vi "Main.vi"() -> ()   [LabVIEW 2012]
uses:
  HeaterConfigurationGlobalAction.ctl
  MFCConfigurationGlobalAction.ctl
  LogActionQueueElement.ctl
  LogAction.ctl
  HardwareActionQueueElement.ctl
  HardwareAction.ctl
  HeaterActionQueueElement.ctl
  HeaterAction.ctl
  MFCActionQueueElement.ctl
  MFCAction.ctl
  <vilib>/Utility/error.llb/DialogType.ctl
  UIActionQueueElement.ctl
  UIAction.ctl
  libs/LV-Utilities/LV-Utilities.lvlib
panel:
  in  "LOGS":bool
  in  "LIVE":bool
  in  "SYSTEM":bool
  in  "DONE":bool
  in  "Tab Control":enum32{"System", "Live", "Logs"}(tab)
  out "MFC Serial Number":string="Serial Number"
  in  "SELECT CONFIG":bool
  out "Setup File":path
  in  "CONFIGURE MFC":bool
  in  "CONFIGURE HEATER":bool
  out "Chamber Name":string="Chamber Name"
  out "Heater Actual Slide":dbl(slide) scale=0.0..200.0 scale format="%#.1f"
  out "Heater Actual (C)":dbl=nan format="%.1f"
  out "Heater Setpoint Slide":dbl(slide) scale=0.0..200.0 scale format="%#.1f"
  out "Heater Setpoint (C)":dbl=nan format="%.1f"
  out "Heater State":enum16{"Not Connected", "Run", "Standby"}(ring)
  out "MFC Actual Slide":dbl(slide) scale=0.0..1000.0 scale format="%#.1f"
  out "MFC Actual (mL/min)":dbl=nan format="%.1f"
  out "MFC Setpoint Slide":dbl(slide) scale=0.0..1000.0 scale format="%#.1f"
  out "MFC Setpoint (mL/min)":dbl=nan format="%.1f"
  out "MFC Valve State":T1(ring)
  out "Live Heater Chart":cluster{"Setpoint (C)":dbl, "Actual (C)":dbl}(graph)
  out "Live MFC Chart":T2(graph)
  in  "CLEAR CHARTS":bool
  out "Heater Setpoint Chart (C)":dbl=nan format="%.1f"
  out "Heater Actual Chart (C)":dbl=nan format="%.1f"
  out "MFC Setpoint Chart (mL/min)":dbl=nan format="%.1f"
  out "MFC Actual Chart (mL/min)":dbl=nan format="%.1f"
  out "MFC Graph":cluster{timestamp[], "Y Data":dbl[]}[](graph)
  out "Heater Graph":cluster{timestamp[], "Y Data":dbl[]}[](graph)
  in  "OPEN LOG":bool
  in  "CLOSE LOG":bool
  out "Opened Log File Path":path
  # "Vacuum Pump"
  # "Config File:"
  # "Actual"
  # "Setpoint"
  # "Actual"
  # "Setpoint"
  # "Heater:"
  # "MFC:"
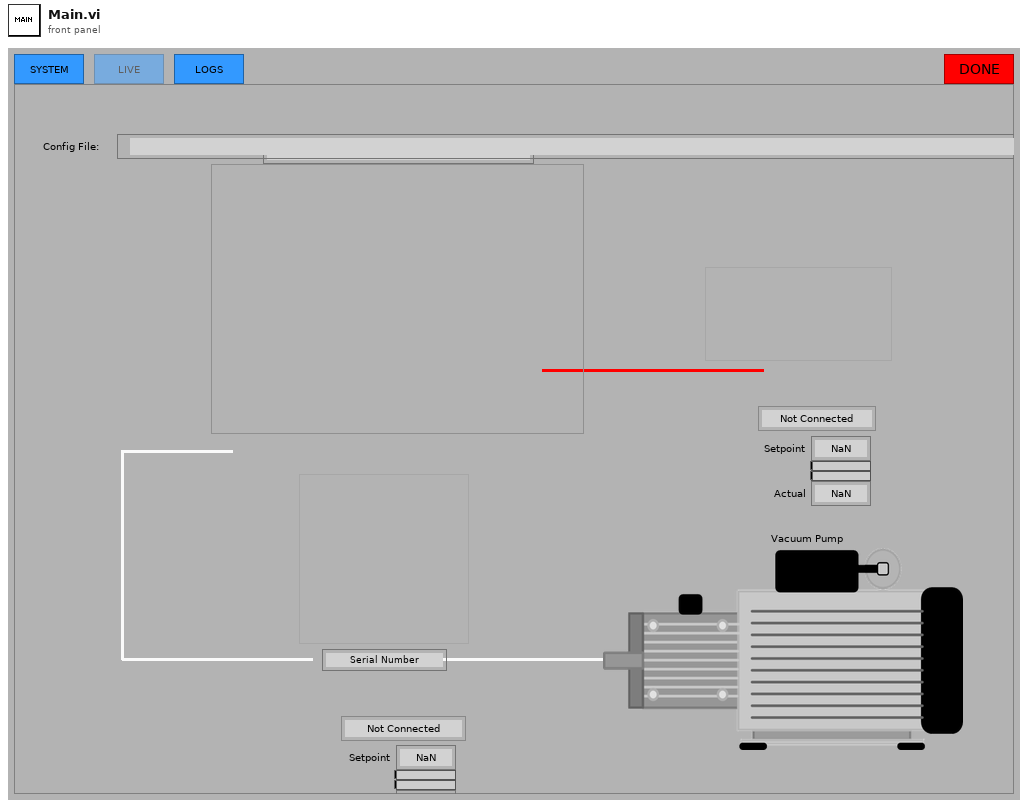
[diagram p1: front panel]
types:
  T1 = enum16{"Not Connected", "Automatic", "Closed", "Purge"}
  T2 = cluster{"Setpoint (mL/min)":dbl, "Actual (mL/min)":dbl}
  T3 = typedef "DataStructures.ctl" = cluster{"Display":refnum<notifier>, "Log":refnum<queue>}
  T4 = typedef "ActionQueues.ctl" = cluster{"UI Action":refnum<queue>, "Hardware Action":refnum<queue>, "Heater Action":refnum<queue>, "MFC Action":refnum<queue>, "Log Action":refnum<queue>}
  T5 = typedef "ExecutableConfiguration.ctl" = cluster{"Default Chamber Folder Path":path, "Default Log Folder Path":path, "Default Monitor":i32, "Center on Monitor?":bool}
  T6 = typedef "MFCActionQueueElement.ctl" = cluster{"Action":T7, "Data":variant}
  T7 = typedef "MFCAction.ctl" = enum16{"Initialize", "Start", "Read", "Write", "Stop", "Error", "Shutdown"}
  T8 = typedef "HeaterActionQueueElement.ctl" = cluster{"Action":T9, "Data":variant}
  T9 = typedef "HeaterAction.ctl" = enum16{"Initialize", "Start", "Read", "Write", "Stop", "Error", "Shutdown"}
  T10 = typedef "HardwareActionQueueElement.ctl" = cluster{"Action":T11, "Data":variant}
  T11 = typedef "HardwareAction.ctl" = enum16{"Initialize", "Collect", "Shutdown"}
  T12 = enum8{"Enabled", "Disabled", "Disabled and Grayed Out"}
  T13 = typedef "LogActionQueueElement.ctl" = cluster{"Action":T14, "Data":variant}
  T14 = typedef "LogAction.ctl" = enum16{"Initialize", "Start", "Log", "Stop", "Error", "Shutdown"}
  T15 = typedef "MFCConfigurationGlobalAction.ctl" = enum16{"Get", "Set", "Reset"}
  T16 = typedef "HeaterConfigurationGlobalAction.ctl" = enum16{"Get", "Set", "Reset"}
  T17 = cluster{"Setpoint (mL/min)":dbl, "Actual (mL/min)":dbl}[]
  T18 = typedef "UIActionQueueElement.ctl" = cluster{"Action":T19, "Data":variant}
  T19 = typedef "UIAction.ctl" = enum16{"Initialize", "Connect", "MFC Connected", "Heater Connected", "Disconnect", "MFC Disconnected", "Heater Disconnected", "Configure MFC", "Configure Heater", "Open Log", "Close Log", "Shutdown"}
  T20 = typedef "Setup.ctl" = cluster{"Chamber Name":string, "Log Folder Path":path, "Heater":T21, "MFC":T22}
  T21 = typedef "HeaterConfiguration.ctl" = cluster{"COM Port":u8, "Setpoint":dbl, "Standby?":bool}
  T22 = typedef "MFCConfiguration.ctl" = cluster{"COM Port":u32, "Timeout (msec)":u32, "Setpoint":dbl, "Valve State":T23, "Gas":T24, "Units":T25, "Serial Number":string, "Firmware Version":string}
  T23 = typedef "Sierra-M100.lvlib/ValveState.ctl" = enum16{"Automatic", "Closed", "Purge"}
  T24 = typedef "Sierra-M100.lvlib/Gas.ctl" = enum16{"Air", "Argon", "CO2", "CO", "Helium", "Hydrogen", "Methane", "Nitrogen", "Nitrous Oxide", "Oxygen"}
  T25 = typedef "Sierra-M100.lvlib/Units.ctl" = enum16{"scc/s", "scc/m", "scc/H", "Ncc/s", "Ncc/m", "Ncc/H", "SCF/s", "SCF/m", "SCF/H", "NM3/s", "NM3/m", "NM3/H", "SM3/s", "SM3/m", "SM3/H", "sl/s", "sl/m", "sl/H", "NL/s", "NL/m", "Nl/H", "g/s", "g/m", "g/H", "kg/s", "kg/m", "kg/H", "lb/s", "lb/m", "lb/H"}
  T26 = typedef "DialogType.ctl" = u16
  T27 = typedef "HardwareDisplayData.ctl" = cluster{"Heater":dbl, "MFC":dbl}
  T28 = typedef "MFCDisplayValveState.ctl" = enum16{"Not Connected", "Automatic", "Closed", "Purge"}
  T29 = typedef "HeaterDisplayState.ctl" = enum16{"Not Connected", "Run", "Standby"}
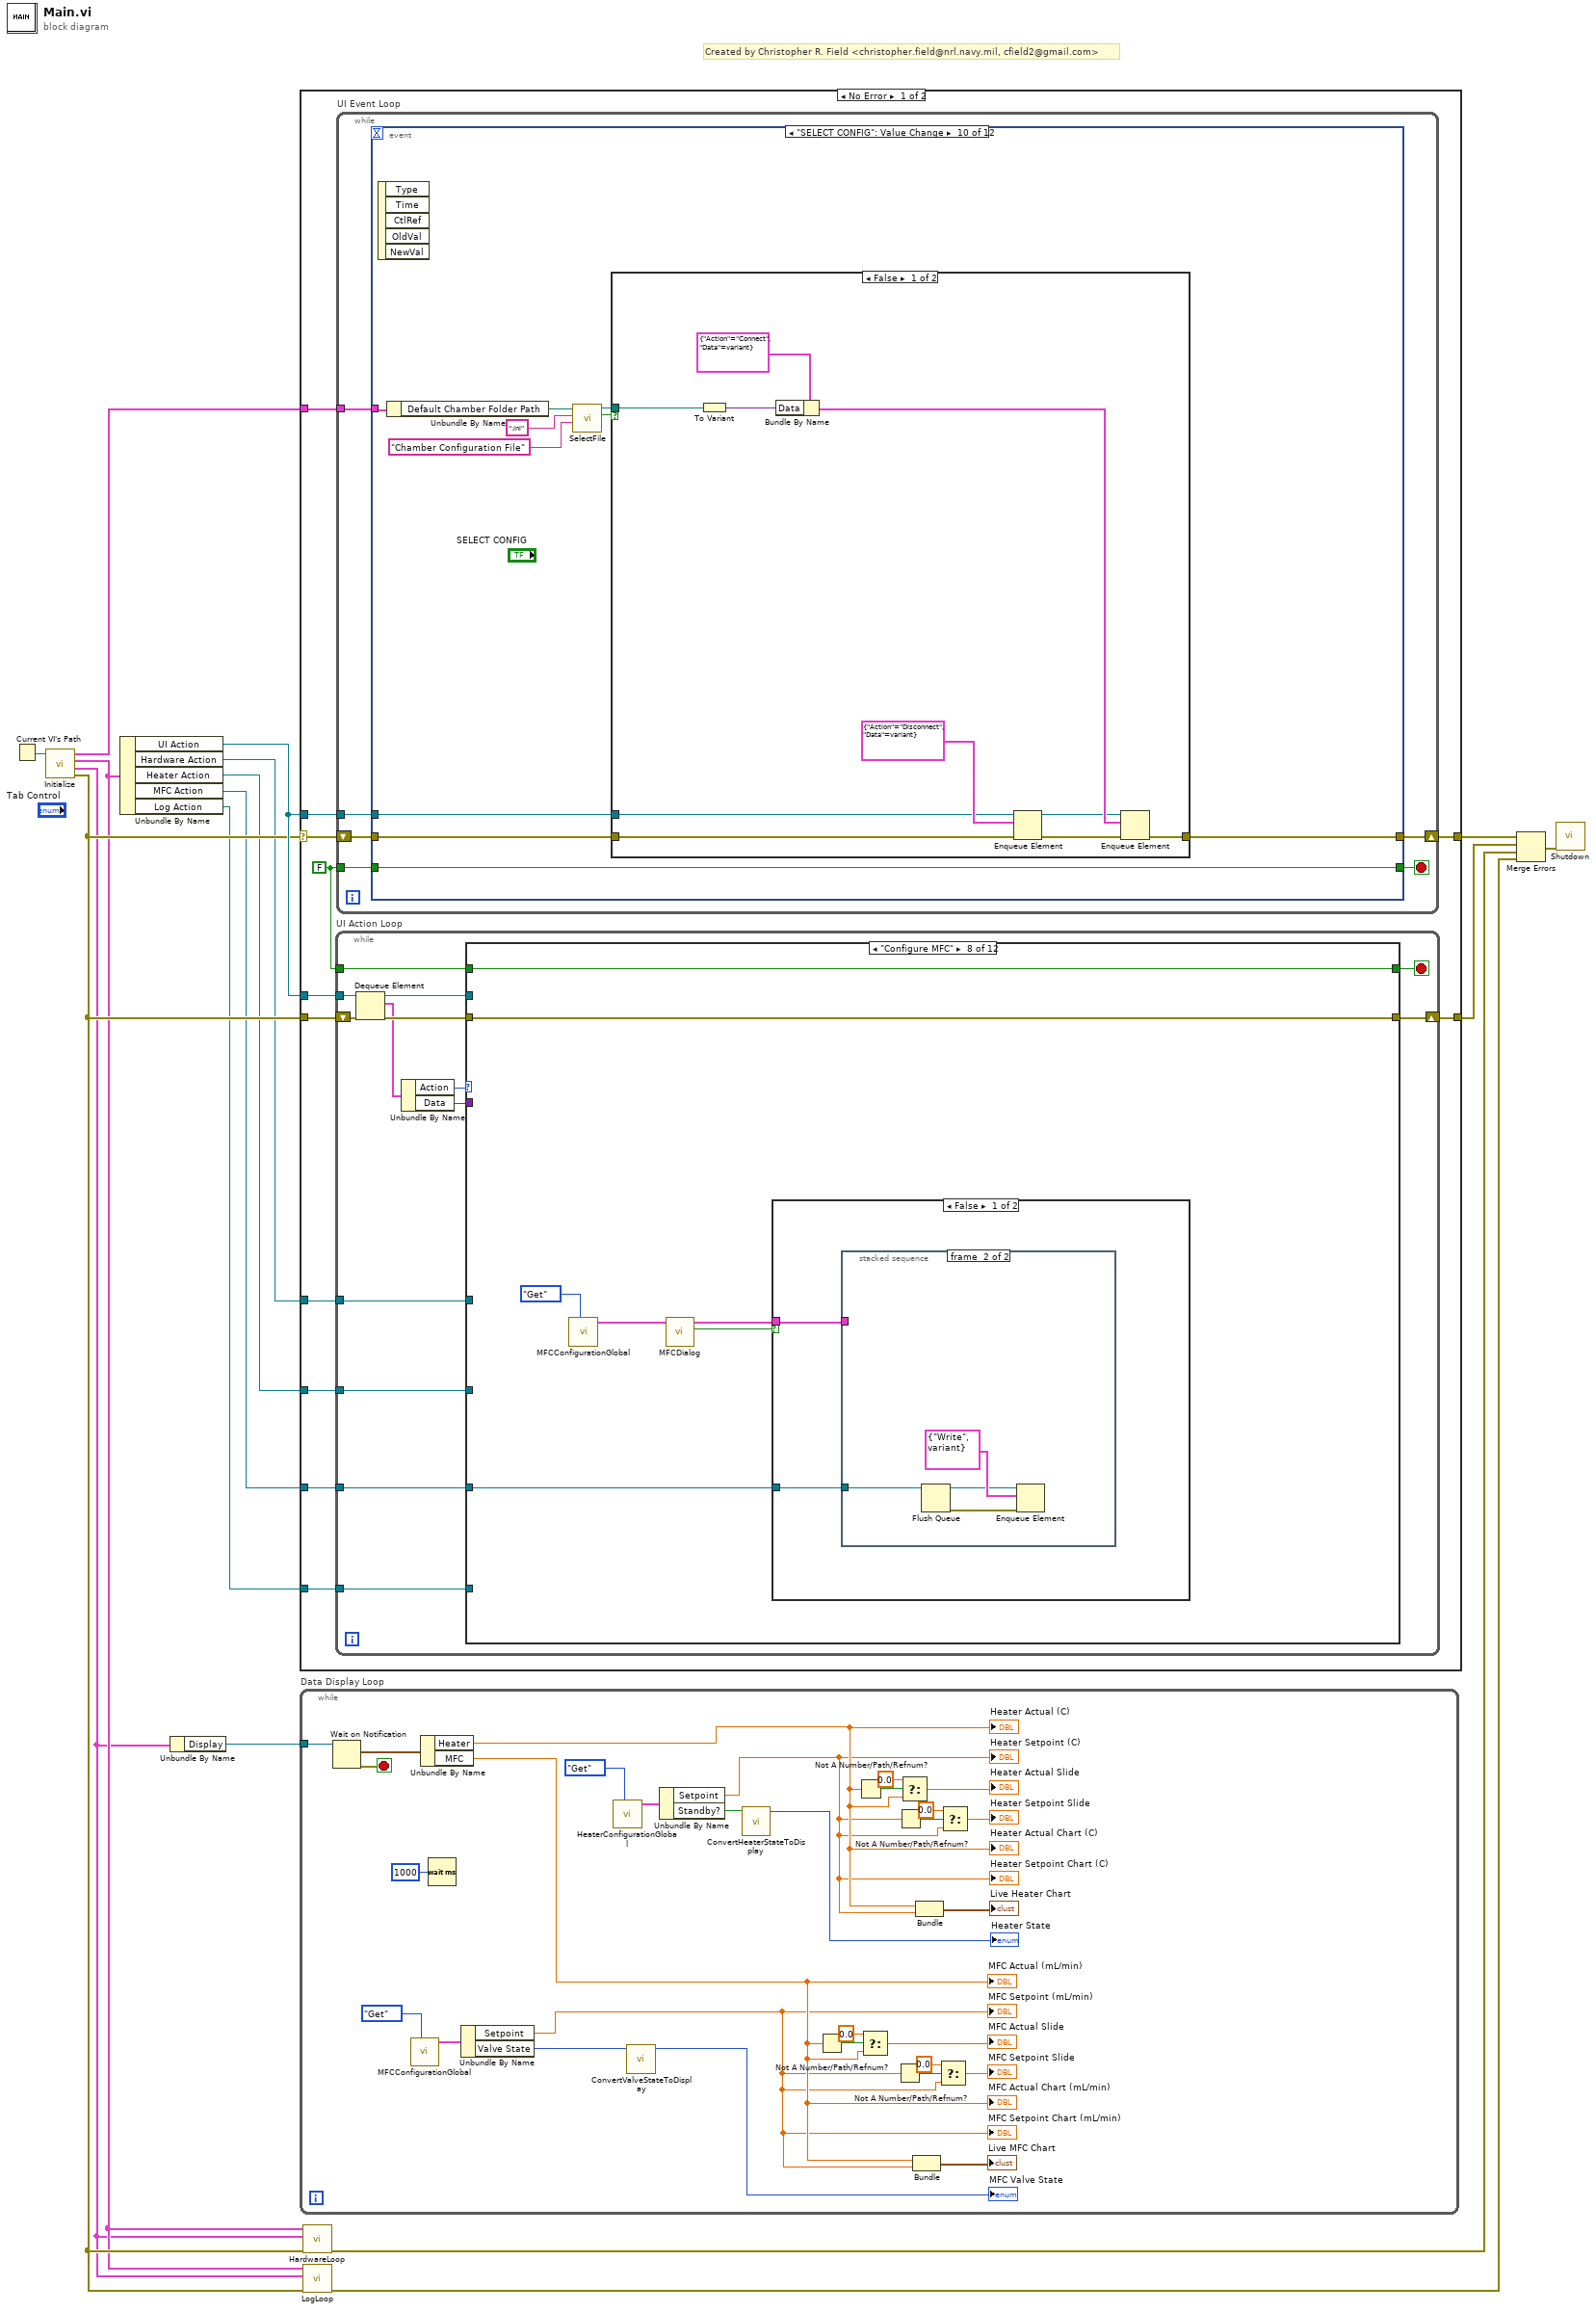
[diagram p0: block diagram]
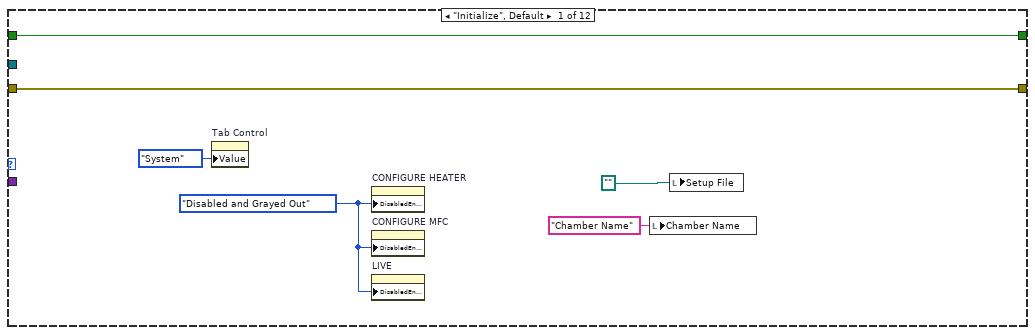
[diagram p2: hidden frame]
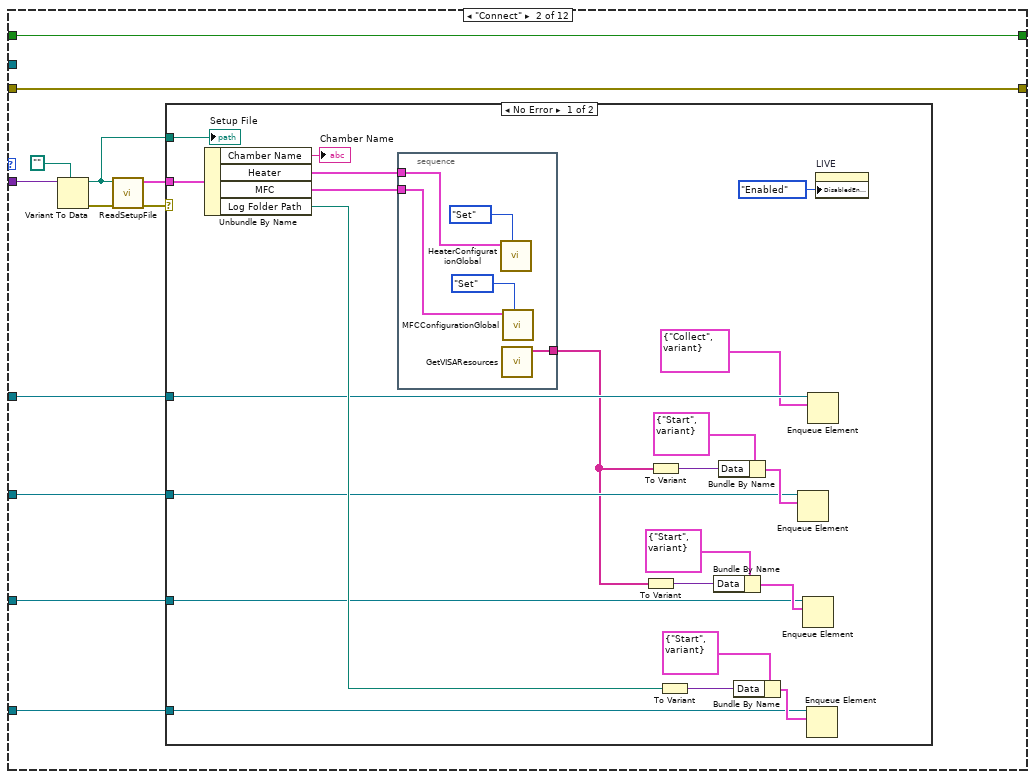
[diagram p3: hidden frame]
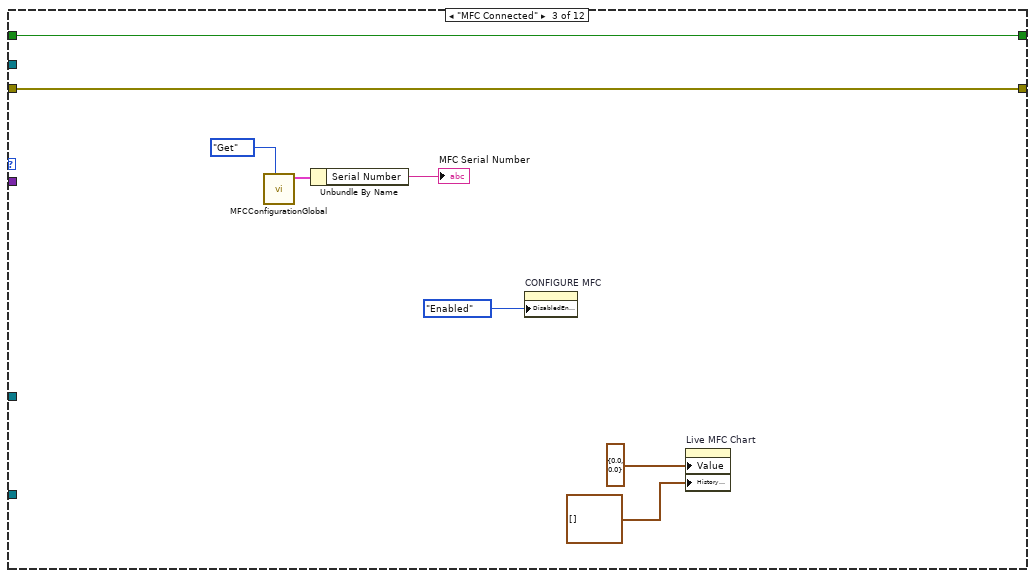
[diagram p5: hidden frame]
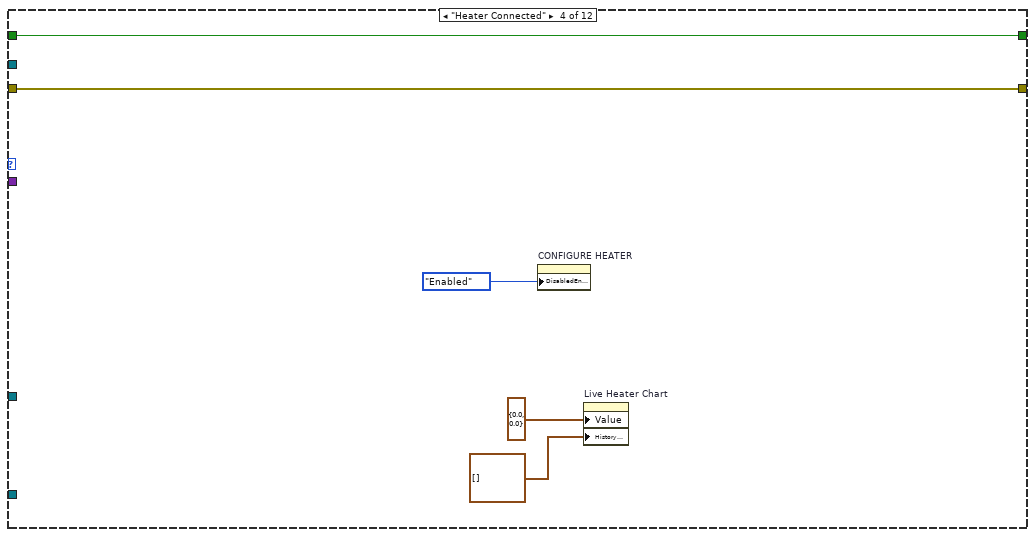
[diagram p6: hidden frame]
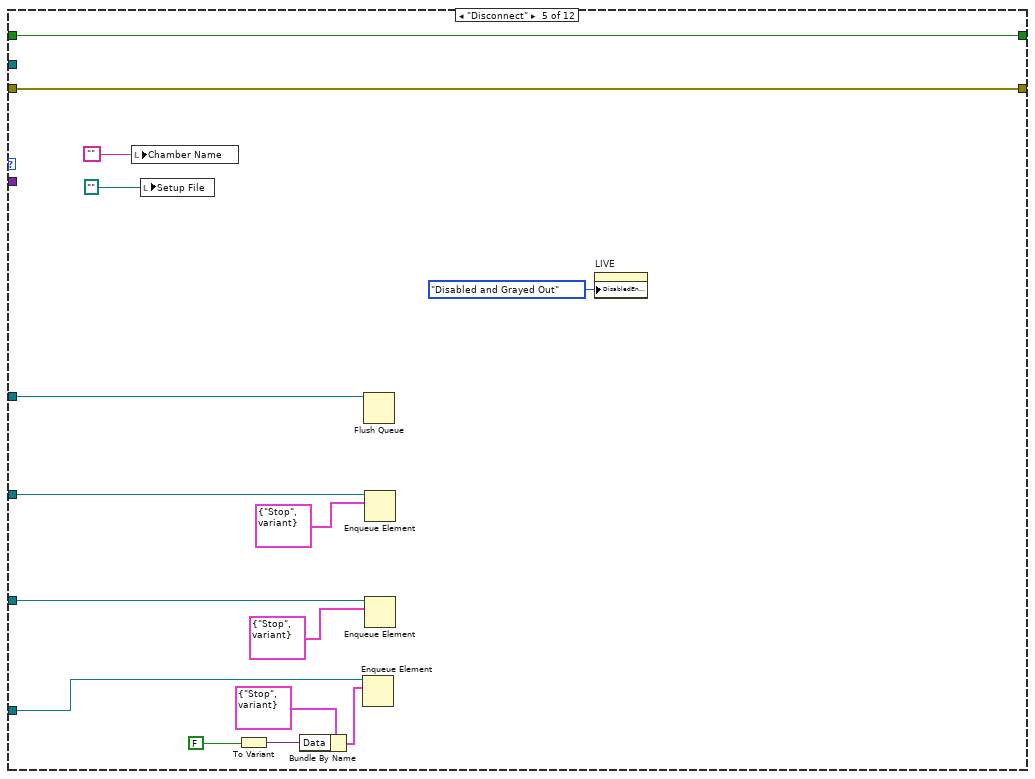
[diagram p7: hidden frame]
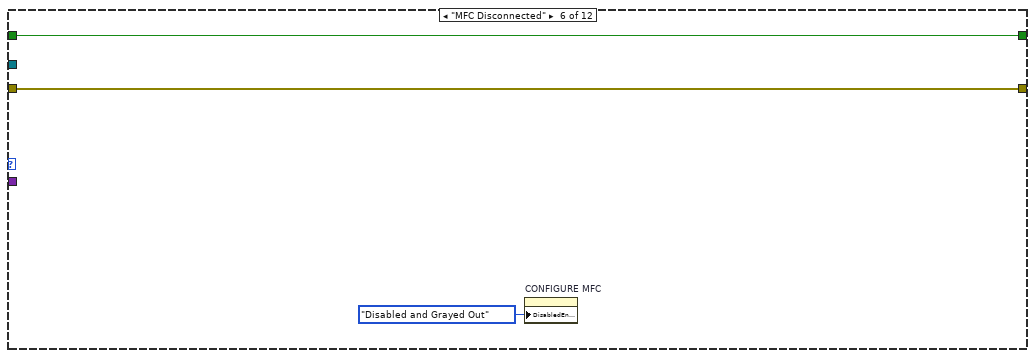
[diagram p8: hidden frame]
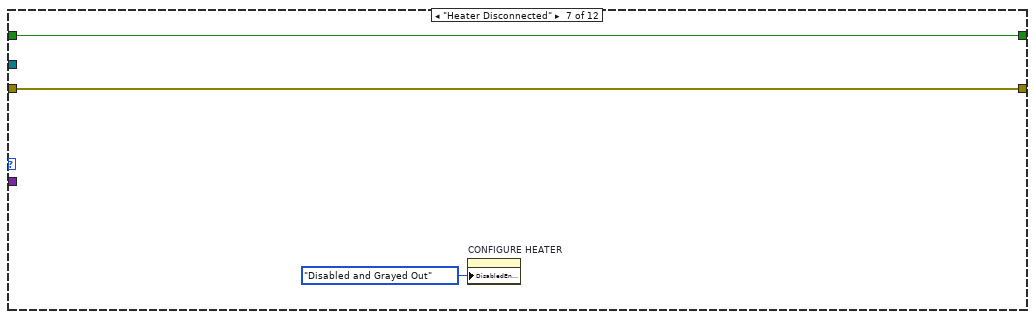
[diagram p9: hidden frame]
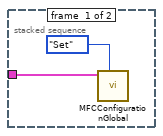
[diagram p10: hidden frame]
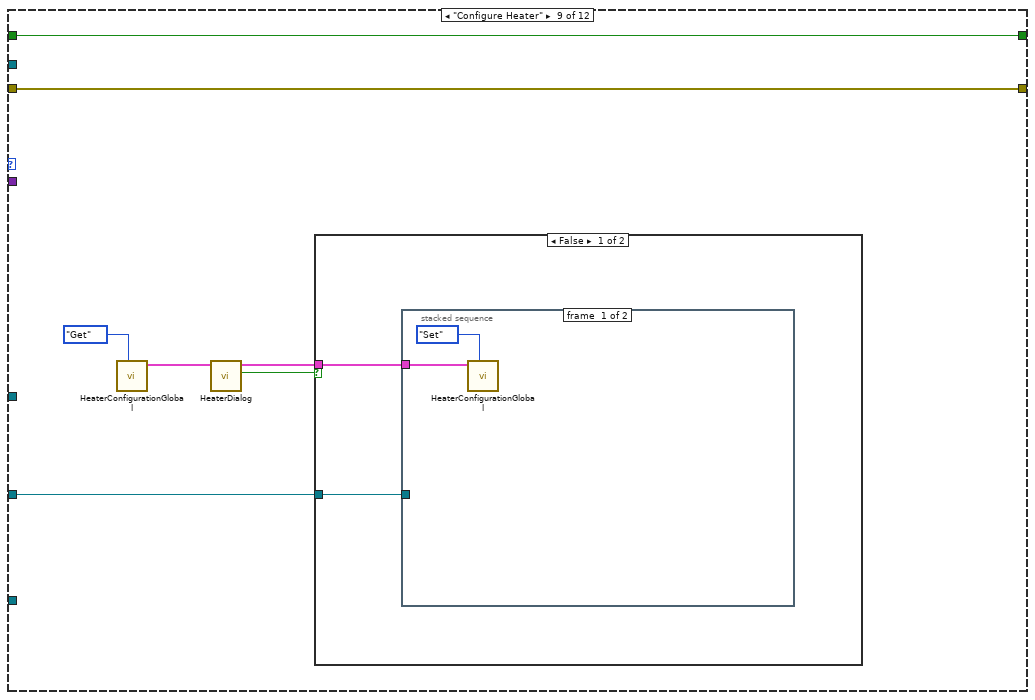
[diagram p12: hidden frame]
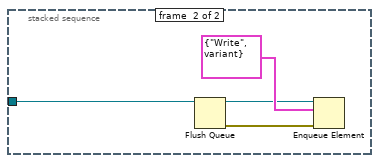
[diagram p13: hidden frame]
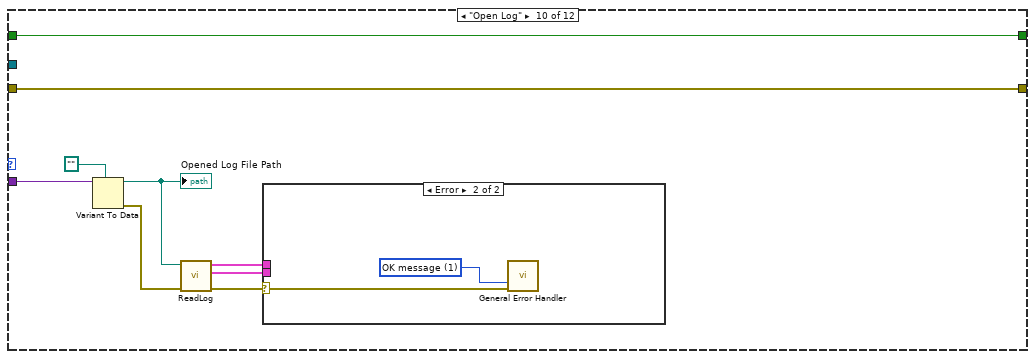
[diagram p15: hidden frame]
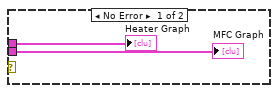
[diagram p16: hidden frame]
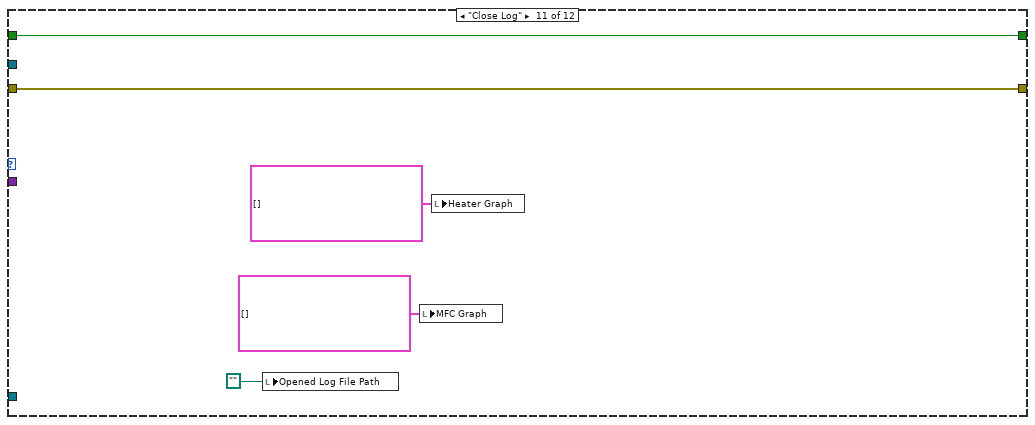
[diagram p17: hidden frame]
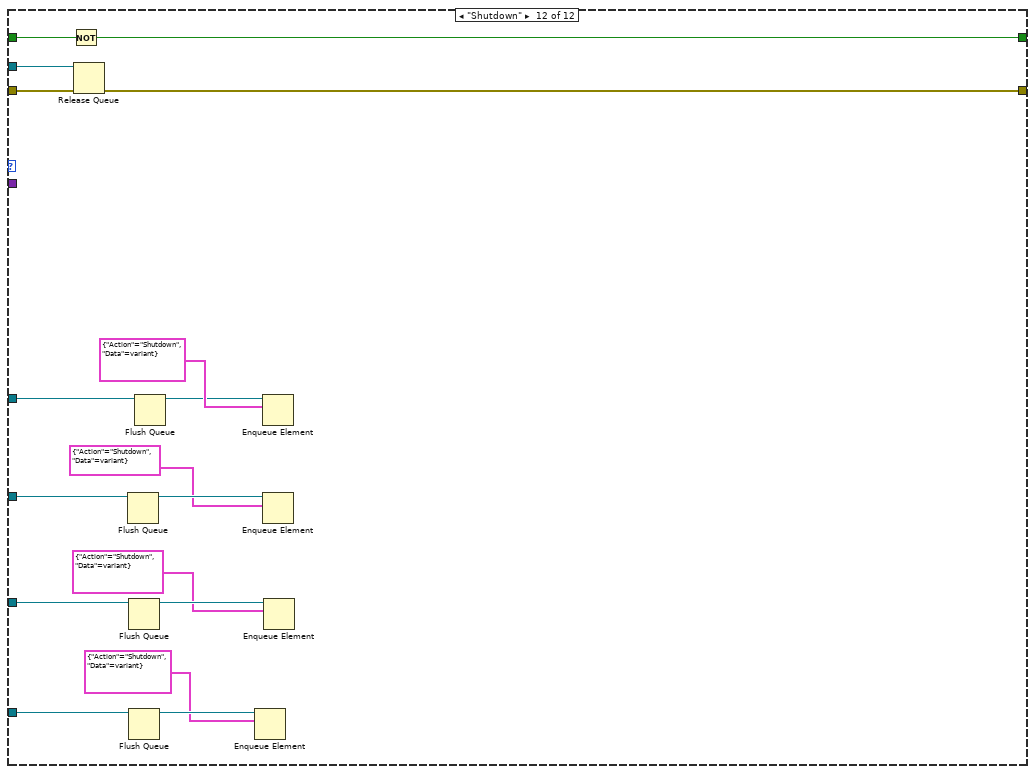
[diagram p18: hidden frame]
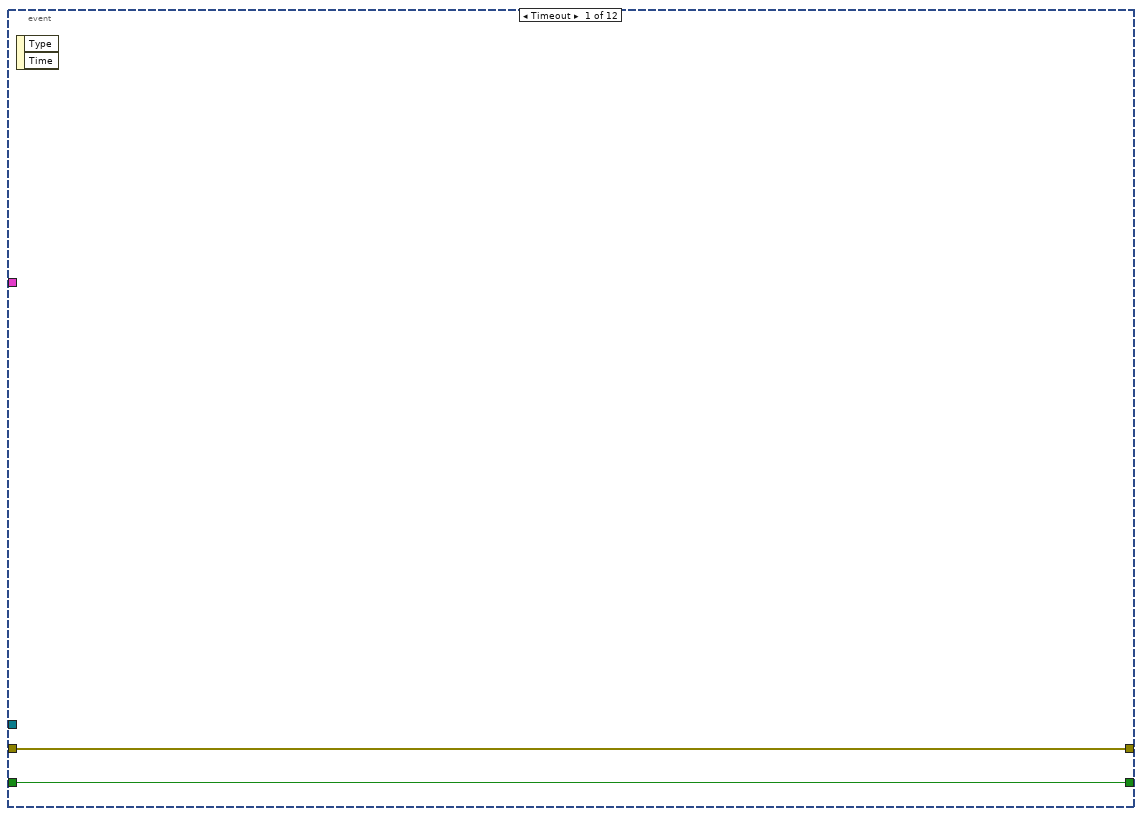
[diagram p19: hidden frame]
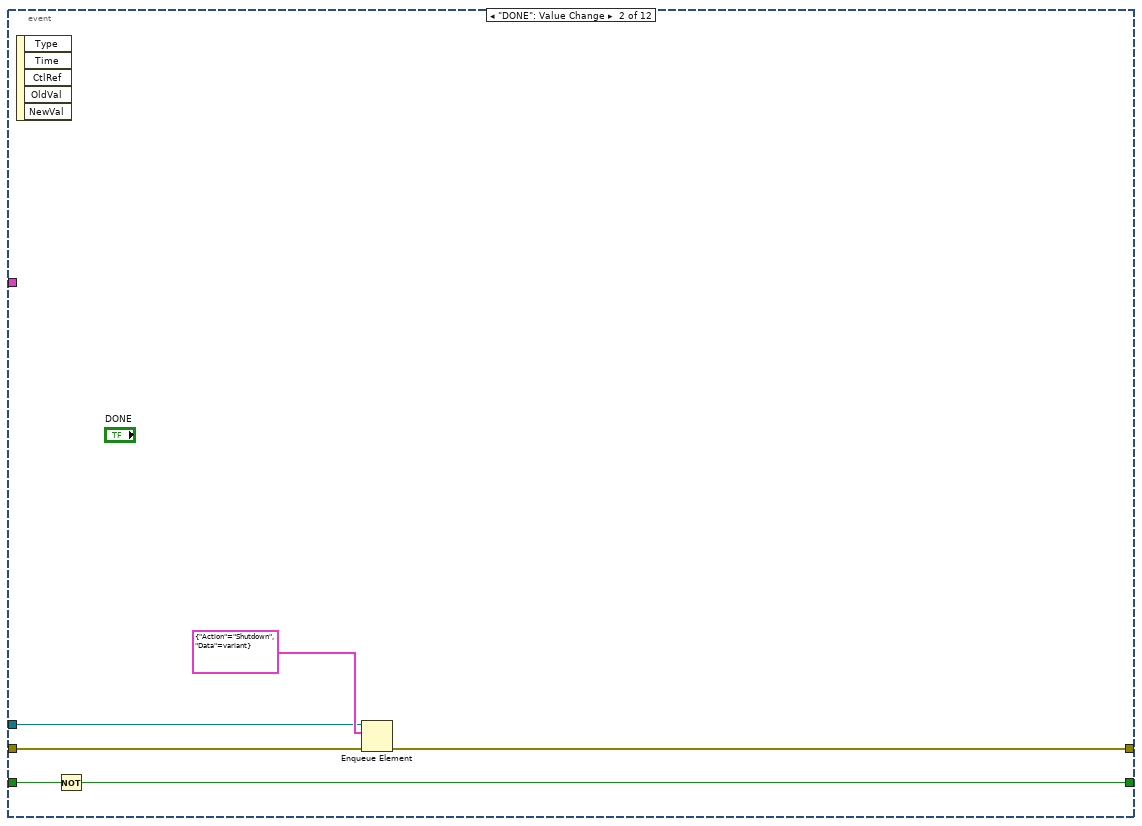
[diagram p20: hidden frame]
diagram:
  # "Created by Christopher R. Field <christopher.field@nrl.navy.mil, cfield2@gmail.com>"
  n1 = Current VI's Path() -> (path=w16:path)
  n2 = call "Initialize.vi"("VI Path"=w16) -> ("Error Out"=w11:errorcluster, "Data Structures"=w6:T3, "Action Queues"=w7:T4, "Executable Configuration"=w4:T5)  [unwired: 7 in]
  n3 = Unbundle By Name(w7) -> ("UI Action"=w15:refnum<queue>, "Hardware Action"=w8:refnum<queue>, "Heater Action"=w3:refnum<queue>, "MFC Action"=w2:refnum<queue>, "Log Action"=w1:refnum<queue>)
  n4 = Unbundle By Name(w6) -> ("Display"=w5:refnum<notifier>)
  n5 = case shown="No Error" w11 {
    selector: w11 -> [w27 w277]
    tunnel: [w28 w277] -> w14
    tunnel: w15 -> [w25 _]
    tunnel: w11 -> [w24 w276]
    tunnel: w15 -> [w23 _]
    tunnel: [w22 w276] -> w13
    tunnel: w8 -> [w21 _]
    tunnel: w4 -> [w20 _]
    tunnel: w3 -> [w19 _]
    tunnel: w2 -> [w18 _]
    tunnel: w1 -> [w17 _]
    frame No Error {
      w26 = FALSE
      n6 = while "UI Action Loop" {
        tunnel: w26 -> [w42]
        tunnel: w25 -> [w32]
        shift-right: [w35] -> w22
        shift-left: w24 -> [w41]
        tunnel: w21 -> [w33]
        tunnel: w19 -> [w31]
        tunnel: w18 -> [w30]
        tunnel: w17 -> [w29]
        stop <- w34 stop-if-true
        n7 = Dequeue Element(queue=w32, error in (no error)=w41) -> (queue out=w40:refnum<queue>, element=w38:T18, error out=w39:errorcluster)  [unwired: 1 in, 1 out]
        n8 = Unbundle By Name(w38) -> ("Action"=w37:T19, "Data"=w36:variant)
        n9 = case shown="\"Configure MFC\"" w37 {
          tunnel: w42 -> [w48 w60 w95 w99 w115 w118 w121 w128 w143 w160 w169 w186]
          tunnel: w40 -> [_ _ _ _ _ _ _ _ _ _ _ w184]
          tunnel: w39 -> [w47 w59 w94 w100 w114 w117 w120 w127 w142 w159 w168 w183]
          tunnel: w36 -> [_ w58 _ _ _ _ _ _ _ w158 _ _]
          tunnel: [w47 w59 w94 w100 w114 w117 w120 w127 w142 w159 w168 w182] -> w35
          tunnel: [w48 w60 w95 w99 w115 w118 w121 w128 w143 w160 w169 w185] -> w34
          tunnel: w33 -> [_ w52 _ _ w101 _ _ _ _ _ _ w171]
          tunnel: w31 -> [_ w51 _ _ w104 _ _ _ w141 _ _ w175]
          tunnel: w30 -> [_ w50 _ _ w103 _ _ w126 _ _ _ w174]
          tunnel: w29 -> [_ w49 _ _ w102 _ _ _ _ _ _ w173]
          frame "Initialize", Default {
            w45 = T12."Disabled and Grayed Out" ("Disabled")
            n10 = property on="Tab Control" class="TabCtl (strict)"("Value"=enum32{"System", "Live", "Logs"}."System" ("Tab Control")) -> ()  [unwired: 2 in, 2 out]
            n11 = property on="CONFIGURE HEATER" class="Bool"("DisabledEnum"=w45) -> ()  [unwired: 2 in, 2 out]
            n12 = property on="CONFIGURE MFC" class="Bool"("DisabledEnum"=w45) -> ()  [unwired: 2 in, 2 out]
            n13 = property on="LIVE" class="Bool"("DisabledEnum"=w45) -> ()  [unwired: 2 in, 2 out]
            n14 = local write "Chamber Name"("Chamber Name" ("Chamber Name")) -> ()
            n15 = local write "Setup File"(path "") -> ()
          }
          frame "Connect" {
            n16 = Variant To Data(type=path "", Variant=w58) -> (data=w53:path, error out=w56:errorcluster)  [unwired: 1 in]
            n17 = call "ReadSetupFile.vi"("Error In"=w56, "Setup File"=w53) -> ("Error Out"=w55:errorcluster, "Setup"=w54:T20)  [unwired: 8 in]
            n18 = case shown="No Error" w55 {
              tunnel: w54 -> [w82 _]
              tunnel: w53 -> [w80 _]
              tunnel: w52 -> [w74 _]
              tunnel: w51 -> [w67 _]
              tunnel: w50 -> [w66 _]
              tunnel: w49 -> [w64 _]
              frame No Error {
                n19 = Unbundle By Name(w82) -> ("Chamber Name"=→"Chamber Name":string, "Heater"=w63:T21, "MFC"=w62:T22, "Log Folder Path"=w77:path)
                n20 = stacked-sequence {
                  tunnel: w63 -> [w86]
                  tunnel: w62 -> [w85]
                  tunnel: [w83] -> w61
                  frame #0 {
                    n21 = call "HeaterConfigurationGlobal.vi"("Action"=HeaterConfigurationGlobalAction."Set", "Set Value"=w86) -> ()  [unwired: 9 in, 1 out]
                    n22 = call "GetVISAResources.vi"() -> ("VISA Resources"=w83:string[])  [unwired: 10 in, 1 out]
                    n23 = call "MFCConfigurationGlobal.vi"("Action"=MFCConfigurationGlobalAction."Set", "Set Value"=w85) -> ()  [unwired: 9 in, 1 out]
                  }
                }
                n24 = To Variant(anything=w61) -> (Variant=w70:variant)
                n25 = To Variant(anything=w61) -> (Variant=w72:variant)
                n26 = To Variant(anything=w77) -> (Variant=w78:variant)
                n27 = Bundle By Name(cluster=T6 {"Action"=enum."Start", "Data"=variant} ("element"), "Data"=w70) -> (w68:T6)
                n28 = Bundle By Name(cluster=T8 {"Action"=enum."Start", "Data"=variant} ("element"), "Data"=w72) -> (w71:T8)
                n29 = Bundle By Name(cluster=T13 {"Action"=enum."Start", "Data"=variant} ("element"), "Data"=w78) -> (w76:T13)
                n30 = Enqueue Element(queue=w67, element=w71) -> ()  [unwired: 2 in, 3 out]
                n31 = Enqueue Element(queue=w66, element=w68) -> ()  [unwired: 2 in, 3 out]
                n32 = Enqueue Element(queue=w64, element=w76) -> ()  [unwired: 2 in, 3 out]
                n33 = Enqueue Element(queue=w74, element=T10 {"Action"=enum."Collect", "Data"=variant}) -> ()  [unwired: 2 in, 3 out]
                n34 = property on="LIVE" class="Bool"("DisabledEnum"=T12."Enabled" ("Disabled")) -> ()  [unwired: 2 in, 2 out]
                "Setup File" <- w80
              }
              frame Error {
              }
            }
          }
          frame "MFC Connected" {
            n35 = call "MFCConfigurationGlobal.vi"("Action"=MFCConfigurationGlobalAction."Get") -> ("Value Out"=w89:T22)  [unwired: 10 in]
            n36 = Unbundle By Name(w89) -> ("Serial Number"=→"MFC Serial Number":string)
            n37 = property on="CONFIGURE MFC" class="Bool"("DisabledEnum"=T12."Enabled" ("Disabled")) -> ()  [unwired: 2 in, 2 out]
            n38 = property on="Live MFC Chart" class="WFChart (strict)"("Value"=T2 {"Setpoint (mL/min)"=0.0, "Actual (mL/min)"=0.0} ("Live MFC Chart"), "History Data"=T17 []) -> ()  [unwired: 2 in, 2 out]
          }
          frame "Heater Connected" {
            n39 = property on="CONFIGURE HEATER" class="Bool"("DisabledEnum"=T12."Enabled" ("Disabled")) -> ()  [unwired: 2 in, 2 out]
            n40 = property on="Live Heater Chart" class="WFChart (strict)"("Value"=cluster{"Setpoint (C)":dbl, "Actual (C)":dbl} {"Setpoint (C)"=0.0, "Actual (C)"=0.0} ("Live Heater Chart"), "History Data"=cluster{"Setpoint (C)":dbl, "Actual (C)":dbl}[] []) -> ()  [unwired: 2 in, 2 out]
          }
          frame "Disconnect" {
            n41 = local write "Chamber Name"("") -> ()
            n42 = local write "Setup File"(path "") -> ()
            n43 = To Variant(anything=FALSE) -> (Variant=w108:variant)
            n44 = Bundle By Name(cluster=T13 {"Action"=enum."Stop", "Data"=variant} ("element"), "Data"=w108) -> (w106:T13)
            n45 = Enqueue Element(queue=w102, element=w106) -> ()  [unwired: 2 in, 3 out]
            n46 = Flush Queue(queue=w101) -> ()  [unwired: 1 in, 3 out]
            n47 = Enqueue Element(queue=w104, element=T8 {"Action"=enum."Stop", "Data"=variant}) -> ()  [unwired: 2 in, 3 out]
            n48 = Enqueue Element(queue=w103, element=T6 {"Action"=enum."Stop", "Data"=variant}) -> ()  [unwired: 2 in, 3 out]
            n49 = property on="LIVE" class="Bool"("DisabledEnum"=T12."Disabled and Grayed Out" ("Disabled")) -> ()  [unwired: 2 in, 2 out]
          }
          frame "MFC Disconnected" {
            n50 = property on="CONFIGURE MFC" class="Bool"("DisabledEnum"=T12."Disabled and Grayed Out" ("Disabled")) -> ()  [unwired: 2 in, 2 out]
          }
          frame "Heater Disconnected" {
            n51 = property on="CONFIGURE HEATER" class="Bool"("DisabledEnum"=T12."Disabled and Grayed Out" ("Disabled")) -> ()  [unwired: 2 in, 2 out]
          }
          frame "Configure MFC" {
            n52 = call "MFCConfigurationGlobal.vi"("Action"=MFCConfigurationGlobalAction."Get") -> ("Value Out"=w124:T22)  [unwired: 10 in]
            n53 = call "MFCDialog.vi"("MFC Configuration In"=w124) -> ("Cancelled?"=w123:bool, "MFC Configuration Out"=w122:T22)  [unwired: 8 in, 1 out]
            n54 = case shown="False" w123 {
              tunnel: w126 -> [w130 _]
              tunnel: w122 -> [w129 _]
              frame False {
                n55 = stacked-sequence {
                  tunnel: w130 -> [_ w133]
                  tunnel: w129 -> [w132 _]
                  frame #0 {
                    n56 = call "MFCConfigurationGlobal.vi"("Action"=MFCConfigurationGlobalAction."Set", "Set Value"=w132) -> ()  [unwired: 9 in, 1 out]
                  }
                  frame #1 {
                    n57 = Flush Queue(queue=w133) -> (queue out=w135:refnum<queue>, error out=w134:errorcluster)  [unwired: 1 in, 1 out]
                    n58 = Enqueue Element(queue=w135, element=T6 {"Action"=enum."Write", "Data"=variant}, error in (no error)=w134) -> ()  [unwired: 1 in, 3 out]
                  }
                }
              }
              frame True {
              }
            }
          }
          frame "Configure Heater" {
            n59 = call "HeaterConfigurationGlobal.vi"("Action"=HeaterConfigurationGlobalAction."Get") -> ("Value Out"=w139:T21)  [unwired: 10 in]
            n60 = call "HeaterDialog.vi"("Heater Configuration In"=w139) -> ("Cancelled?"=w138:bool, "Heater Configuration Out"=w137:T21)  [unwired: 8 in, 1 out]
            n61 = case shown="False" w138 {
              tunnel: w141 -> [w145 _]
              tunnel: w137 -> [w144 _]
              frame False {
                n62 = stacked-sequence {
                  tunnel: w145 -> [_ w148]
                  tunnel: w144 -> [w147 _]
                  frame #0 {
                    n63 = call "HeaterConfigurationGlobal.vi"("Action"=HeaterConfigurationGlobalAction."Set", "Set Value"=w147) -> ()  [unwired: 9 in, 1 out]
                  }
                  frame #1 {
                    n64 = Flush Queue(queue=w148) -> (queue out=w150:refnum<queue>, error out=w149:errorcluster)  [unwired: 1 in, 1 out]
                    n65 = Enqueue Element(queue=w150, element=T8 {"Action"=enum."Write", "Data"=variant}, error in (no error)=w149) -> ()  [unwired: 1 in, 3 out]
                  }
                }
              }
              frame True {
              }
            }
          }
          frame "Open Log" {
            n66 = Variant To Data(type=path "", Variant=w158) -> (data=w156:path, error out=w152:errorcluster)  [unwired: 1 in]
            "Opened Log File Path" <- w156
            n67 = call "ReadLog.vi"("Error In"=w152, "Log File Path"=w156) -> ("Error Out"=w155:errorcluster, "MFC Plots"=w153:cluster{timestamp[], "Y Data":dbl[]}[], "Heater Plots"=w154:cluster{timestamp[], "Y Data":dbl[]}[])  [unwired: 7 in]
            n68 = case shown="Error" w155 {
              selector: w155 -> [_ w164]
              tunnel: w154 -> [w162 _]
              tunnel: w153 -> [w161 _]
              frame No Error {
                "Heater Graph" <- w162
                "MFC Graph" <- w161
              }
              frame Error {
                w163 = T26 1 items=["no dialog", "OK message", "continue or stop message", "OK message + warnings", "continue/stop + warnings"] ("type of dialog (OK msg:1)")
                n69 = call <vilib>:"General Error Handler.vi"("type of dialog (OK msg:1)"=w163, "error in (no error)"=w164) -> ()  [unwired: 9 in, 5 out]
              }
            }
          }
          frame "Close Log" {
            n70 = local write "Opened Log File Path"(path "") -> ()
            n71 = local write "MFC Graph"(cluster{timestamp[], "Y Data":dbl[]}[] [] ("MFC Graph")) -> ()
            n72 = local write "Heater Graph"(cluster{timestamp[], "Y Data":dbl[]}[] [] ("Heater Graph")) -> ()
          }
          frame "Shutdown" {
            n73 = Not(x=w186) -> (.not. x?=w185:bool)
            n74 = Release Queue(queue=w184, error in (no error)=w183) -> (error out=w182:errorcluster)  [unwired: 1 in, 2 out]
            n75 = Flush Queue(queue=w175) -> (queue out=w181:refnum<queue>)  [unwired: 1 in, 2 out]
            n76 = Flush Queue(queue=w174) -> (queue out=w179:refnum<queue>)  [unwired: 1 in, 2 out]
            n77 = Flush Queue(queue=w173) -> (queue out=w177:refnum<queue>)  [unwired: 1 in, 2 out]
            n78 = Flush Queue(queue=w171) -> (queue out=w170:refnum<queue>)  [unwired: 1 in, 2 out]
            n79 = Enqueue Element(queue=w177, element=T13 {"Action"=enum."Shutdown", "Data"=variant}) -> ()  [unwired: 2 in, 3 out]
            n80 = Enqueue Element(queue=w170, element=T10 {"Action"=enum."Shutdown", "Data"=variant}) -> ()  [unwired: 2 in, 3 out]
            n81 = Enqueue Element(queue=w181, element=T8 {"Action"=enum."Shutdown", "Data"=variant}) -> ()  [unwired: 2 in, 3 out]
            n82 = Enqueue Element(queue=w179, element=T6 {"Action"=enum."Shutdown", "Data"=variant}) -> ()  [unwired: 2 in, 3 out]
          }
        }
      }
      n83 = while "UI Event Loop" {
        tunnel: w26 -> [w192]
        shift-right: [w189] -> w28
        shift-left: w27 -> [w190]
        tunnel: w23 -> [w188]
        tunnel: w20 -> [w187]
        stop <- w191 stop-if-true
        n84 = event shown="[9] \"SELECT CONFIG\": Value Change" {
          selector: _ -> [_ _ _ _ _ _ _ _ _ _ _ _]
          dyn-events: _ -> [_ _ _ _ _ _ _ _ _ _ _ _]
          timeout: _ -> [_ _ _ _ _ _ _ _ _ _ _ _]
          tunnel: w192 -> [w194 w200 w206 w209 w211 w214 w220 w225 w231 w241 w262 w275]
          tunnel: [w194 w199 w205 w209 w211 w214 w220 w225 w231 w241 w262 w275] -> w191
          tunnel: w190 -> [w193 w198 w203 w207 w210 w213 w219 w224 w230 w236 w256 w274]
          tunnel: [w193 w197 w202 w207 w210 w213 w218 w223 w230 w235 w255 w273] -> w189
          tunnel: w188 -> [_ w195 w201 _ _ _ w216 w221 _ w237 w257 w271]
          tunnel: w187 -> [_ _ _ _ _ _ _ _ _ w232 w253 _]
          event Timeout {
            n85 = event-data() -> ()  [unwired: 1 in, 2 out]
          }
          event "DONE": Value Change {
            n86 = event-data() -> ()  [unwired: 1 in, 5 out]
            n87 = Not(x=w200) -> (.not. x?=w199:bool)
            n88 = Enqueue Element(queue=w195, element=T18 {"Action"=enum."Shutdown", "Data"=variant}, error in (no error)=w198) -> (error out=w197:errorcluster)  [unwired: 1 in, 2 out]
          }
          event Panel Close? {
            n89 = event-data() -> ()  [unwired: 1 in, 3 out]
            n90 = Not(x=w206) -> (.not. x?=w205:bool)
            n91 = Enqueue Element(queue=w201, element=T18 {"Action"=enum."Shutdown", "Data"=variant}, error in (no error)=w203) -> (error out=w202:errorcluster)  [unwired: 1 in, 2 out]
            n92 = event-data("Discard?"=w205) -> ()  [unwired: 1 in, 1 out]
          }
          event "SYSTEM": Value Change {
            n93 = event-data() -> ()  [unwired: 1 in, 5 out]
            n94 = property on="Tab Control" class="TabCtl (strict)"("Value"=enum32{"System", "Live", "Logs"}."System" ("Tab Control")) -> ()  [unwired: 2 in, 2 out]
          }
          event "LIVE": Value Change {
            n95 = event-data() -> ()  [unwired: 1 in, 5 out]
            n96 = property on="Tab Control" class="TabCtl (strict)"("Value"=enum32{"System", "Live", "Logs"}."Live" ("Tab Control")) -> ()  [unwired: 2 in, 2 out]
          }
          event "LOGS": Value Change {
            n97 = event-data() -> ()  [unwired: 1 in, 5 out]
            n98 = property on="Tab Control" class="TabCtl (strict)"("Value"=enum32{"System", "Live", "Logs"}."Logs" ("Tab Control")) -> ()  [unwired: 2 in, 2 out]
          }
          event "CONFIGURE HEATER": Value Change {
            n99 = event-data() -> ()  [unwired: 1 in, 5 out]
            n100 = Enqueue Element(queue=w216, element=T18 {"Action"=enum."Configure Heater", "Data"=variant}, error in (no error)=w219) -> (error out=w218:errorcluster)  [unwired: 1 in, 2 out]
          }
          event "CONFIGURE MFC": Value Change {
            n101 = event-data() -> ()  [unwired: 1 in, 5 out]
            n102 = Enqueue Element(queue=w221, element=T18 {"Action"=enum."Configure MFC", "Data"=variant}, error in (no error)=w224) -> (error out=w223:errorcluster)  [unwired: 1 in, 2 out]
          }
          event "CLEAR CHARTS": Value Change {
            n103 = event-data() -> ()  [unwired: 1 in, 5 out]
            n104 = property on="Live Heater Chart" class="WFChart (strict)"("Value"=cluster{"Setpoint (C)":dbl, "Actual (C)":dbl} {"Setpoint (C)"=0.0, "Actual (C)"=0.0} ("Live Heater Chart"), "History Data"=cluster{"Setpoint (C)":dbl, "Actual (C)":dbl}[] []) -> ()  [unwired: 2 in, 2 out]
            n105 = property on="Live MFC Chart" class="WFChart (strict)"("Value"=T2 {"Setpoint (mL/min)"=0.0, "Actual (mL/min)"=0.0} ("Live MFC Chart"), "History Data"=T17 []) -> ()  [unwired: 2 in, 2 out]
          }
          event "SELECT CONFIG": Value Change {
            n106 = event-data() -> ()  [unwired: 1 in, 5 out]
            n107 = Unbundle By Name(w232) -> ("Default Chamber Folder Path"=w233:path)
            n108 = call "SelectFile.vi"("File Description"="Chamber Configuration File", "File Extension (.*)"=".ini", "Start Path"=w233) -> ("Cancelled?"=w238:bool, "Selected File Path"=w234:path)  [unwired: 6 in, 1 out]
            n109 = case shown="False" w238 {
              tunnel: w237 -> [w242 _]
              tunnel: w236 -> [w246 w252]
              tunnel: [w251 w252] -> w235
              tunnel: w234 -> [w248 _]
              frame False {
                n110 = To Variant(anything=w248) -> (Variant=w249:variant)
                n111 = Bundle By Name(cluster=T18 {"Action"=enum."Connect", "Data"=variant} ("element"), "Data"=w249) -> (w247:T18)
                n112 = Enqueue Element(queue=w242, element=T18 {"Action"=enum."Disconnect", "Data"=variant}, error in (no error)=w246) -> (queue out=w244:refnum<queue>, error out=w245:errorcluster)  [unwired: 1 in, 1 out]
                n113 = Enqueue Element(queue=w244, element=w247, error in (no error)=w245) -> (error out=w251:errorcluster)  [unwired: 1 in, 2 out]
              }
              frame True {
              }
            }
          }
          event "OPEN LOG": Value Change {
            n114 = event-data() -> ()  [unwired: 1 in, 5 out]
            n115 = Unbundle By Name(w253) -> ("Default Log Folder Path"=w254:path)
            n116 = call "SelectFile.vi"("File Description"="Sample Chamber Log File", "File Extension (.*)"=".log", "Start Path"=w254) -> ("Cancelled?"=w259:bool, "Selected File Path"=w258:path)  [unwired: 6 in, 1 out]
            n117 = case shown="False" w259 {
              tunnel: w258 -> [w264 _]
              tunnel: w257 -> [w263 _]
              tunnel: w256 -> [w269 w270]
              tunnel: [w268 w270] -> w255
              frame False {
                n118 = To Variant(anything=w264) -> (Variant=w265:variant)
                n119 = Bundle By Name(cluster=T18 {"Action"=enum."Open Log", "Data"=variant} ("element"), "Data"=w265) -> (w266:T18)
                n120 = Enqueue Element(queue=w263, element=w266, error in (no error)=w269) -> (error out=w268:errorcluster)  [unwired: 1 in, 2 out]
              }
              frame True {
              }
            }
          }
          event "CLOSE LOG": Value Change {
            n121 = event-data() -> ()  [unwired: 1 in, 5 out]
            n122 = Enqueue Element(queue=w271, element=T18 {"Action"=enum."Close Log", "Data"=variant}, error in (no error)=w274) -> (error out=w273:errorcluster)  [unwired: 1 in, 2 out]
          }
        }
      }
    }
    frame Error {
    }
  }
  n123 = while "Data Display Loop" {
    tunnel: w5 -> [w292]
    stop <- w307 stop-if-true
    n124 = Wait on Notification(notifier=w292) -> (notification=w293:T27, error out=w307:errorcluster)  [unwired: 3 in, 2 out]
    n125 = call "MFCConfigurationGlobal.vi"("Action"=MFCConfigurationGlobalAction."Get") -> ("Value Out"=w283:T22)  [unwired: 10 in]
    n126 = Unbundle By Name(w293) -> ("Heater"=w291:dbl, "MFC"=w290:dbl)
    "Heater Actual (C)" <- w291
    "Heater Actual Chart (C)" <- w291
    "MFC Actual Chart (mL/min)" <- w290
    "MFC Actual (mL/min)" <- w290
    n127 = Wait (ms)(milliseconds to wait=u32 1000) -> ()  [unwired: 1 out]
    n128 = Unbundle By Name(w283) -> ("Setpoint"=w279:dbl, "Valve State"=w281:T23)
    "MFC Setpoint Chart (mL/min)" <- w279
    "MFC Setpoint (mL/min)" <- w279
    n129 = call "HeaterConfigurationGlobal.vi"("Action"=HeaterConfigurationGlobalAction."Get") -> ("Value Out"=w288:T21)  [unwired: 10 in]
    n130 = call "ConvertValveStateToDisplay.vi"("Valve State"=w281) -> ("MFC Valve State"=→"MFC Valve State":T28)  [unwired: 10 in]
    n131 = Unbundle By Name(w288) -> ("Setpoint"=w287:dbl, "Standby?"=w286:bool)
    "Heater Setpoint Chart (C)" <- w287
    "Heater Setpoint (C)" <- w287
    n132 = call "ConvertHeaterStateToDisplay.vi"("Standby?"=w286) -> ("Heater Display State"=→"Heater State":T29)  [unwired: 10 in]
    n133 = Not A Number/Path/Refnum?(number/path/refnum=w290) -> (NaN/Path/Refnum?=w294:bool)
    n134 = Not A Number/Path/Refnum?(number/path/refnum=w291) -> (NaN/Path/Refnum?=w306:bool)
    n135 = Select(t=0.0, s=w294, f=w290) -> (s? t:f=→"MFC Actual Slide":dbl)
    n136 = Not A Number/Path/Refnum?(number/path/refnum=w279) -> (NaN/Path/Refnum?=w297:bool)
    n137 = Not A Number/Path/Refnum?(number/path/refnum=w287) -> (NaN/Path/Refnum?=w304:bool)
    n138 = Select(t=0.0, s=w306, f=w291) -> (s? t:f=→"Heater Actual Slide":dbl)
    n139 = Bundle("MFC"=w290, "Setpoint"=w279) -> (→"Live MFC Chart":cluster{"MFC":dbl, "Setpoint":dbl})  [unwired: 1 in]
    n140 = Bundle("Heater"=w291, "Setpoint"=w287) -> (→"Live Heater Chart":cluster{"Heater":dbl, "Setpoint":dbl})  [unwired: 1 in]
    n141 = Select(t=0.0, s=w297, f=w279) -> (s? t:f=→"MFC Setpoint Slide":dbl)
    n142 = Select(t=0.0, s=w304, f=w287) -> (s? t:f=→"Heater Setpoint Slide":dbl)
  }
  n143 = call "HardwareLoop.vi"("Error In"=w11, "Data Structures"=w6, "Action Queues"=w7) -> ("Error Out"=w10:errorcluster)  [unwired: 8 in]
  n144 = call "LogLoop.vi"("Error In"=w11, "Data Structures"=w6, "Action Queues"=w7) -> ("Error Out"=w9:errorcluster)  [unwired: 8 in]
  n145 = Merge Errors(w14, w13, w10, w9) -> (w12:errorcluster)
  n146 = call "Shutdown.vi"("Error In"=w12) -> ()  [unwired: 11 in]
